vi "network_ping.vi"() -> ()   [LabVIEW 2011]
doc: "Use this template to build a standard state machine design pattern. Each state executes code and determines which state to transition to. Contrast this design pattern with the User Interface Event Handler pattern, in which code executes in response to user actions. Contrast this design pattern also with the Queued Message Handler pattern, in which each message handling code can queue zero or more new messages."
uses:
  StateMachineStates_ping.ctl
panel:
  out "RoundtripTime":i64
  out "Status":i32(ring) items=["Success"=0, "DestinationNetworkUnreachable"=11002, "DestinationHostUnreachable"=11003, "DestinationProhibited, DestinationProtocolUnreachable"=11004, "DestinationPortUnreachable"=11005, "NoResources"=11006, "BadOption"=11007, "HardwareError"=11008, "PacketTooBig"=11009, "TimedOut"=11010, "BadRoute"=11012, "TtlExpired"=11013, "TtlReassemblyTimeExceeded"=11014, "ParameterProblem"=11015, "SourceQuench"=11016, "BadDestination"=11018, "DestinationUnreachable"=11040, "TimeExceeded"=11041, "BadHeader"=11042, "UnrecognizedNextHeader"=11043, "IcmpError"=11044, "DestinationScopeMismatch"=11045, "Unknown"=-1]
  in  "hostNameOrAddress":string="127.0.0.1"
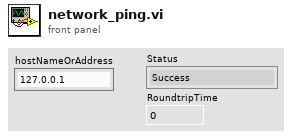
[diagram p1: front panel]
types:
  T1 = typedef "StateMachineStates_ping.ctl" = enum16{"Initialize", "ping_ok", "no_ping", "email", "Stop"}
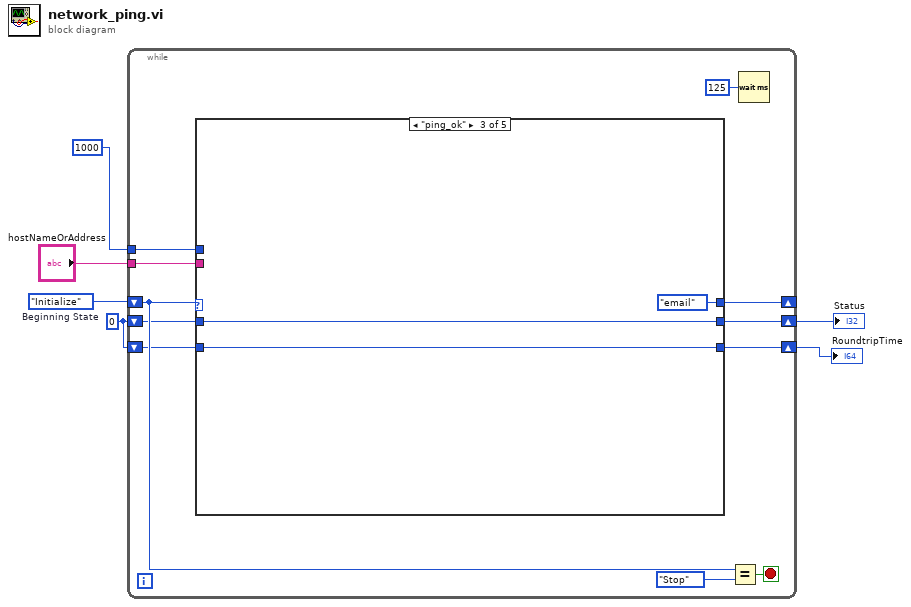
[diagram p0: block diagram]
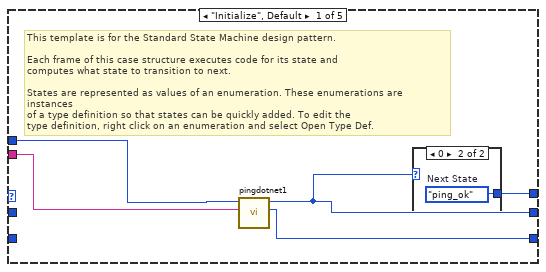
[diagram p2: hidden frame]
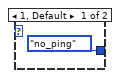
[diagram p3: hidden frame]
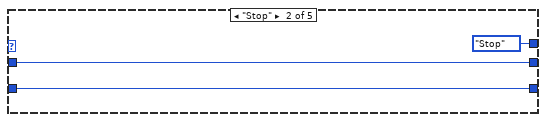
[diagram p4: hidden frame]
diagram:
  w1 = 0 ("Status")
  w6 = StateMachineStates_ping."Initialize"  # Beginning State
  n1 = while {
    shift-right: [w14] -> _
    shift-left: w6 -> [w15]
    tunnel: 1000 ("timeout") -> [w12]
    tunnel: "hostNameOrAddress" -> [w11]
    shift-right: [w10] -> w3
    shift-left: w1 -> [w9]
    shift-right: [w8] -> w2
    shift-left: w1 -> [w7]
    stop <- w17 stop-if-true
    n2 = case shown="\"ping_ok\"" w15 {
      tunnel: [w22 StateMachineStates_ping."Stop" ("Next State") StateMachineStates_ping."email" ("Next State") _ _] -> w14
      tunnel: w12 -> [w21 _ _ _ _]
      tunnel: w11 -> [w20 _ _ _ _]
      tunnel: [w18 w26 w29 _ _] -> w10
      tunnel: w9 -> [_ w26 w29 _ _]
      tunnel: [w19 w25 w30 _ _] -> w8
      tunnel: w7 -> [_ w25 w30 _ _]
      frame "Initialize", Default {
        # "This template is for the Standard State Machine design pattern.\n\nEach frame of this case structure executes code for its state and\ncomputes what state to transition to next.\n\nStates are represented as values of an enumeration. These enumerations are instances\nof a type definition so that states can be quickly added. To edit the \ntype definition, right click on an enumeration and select Open Type Def."
        n3 = call "pingdotnet1.vi"("hostNameOrAddress"=w20, "timeout"=w21) -> ("RoundtripTime"=w19:i64, "Status"=w18:i32)  [unwired: 4 in]
        n4 = case shown="0" w18 {
          tunnel: [StateMachineStates_ping."no_ping" ("Next State") w24] -> w22
          frame 1, Default {
          }
          frame 0 {
            w24 = StateMachineStates_ping."ping_ok"  # Next State
          }
        }
      }
      frame "Stop" {
      }
      frame "ping_ok" {
      }
      frame "no_ping" {
      }
      frame "email" {
      }
    }
    n5 = Equal?(x=w15, y=StateMachineStates_ping."Stop" ("States")) -> (x = y?=w17:bool)
    n6 = Wait (ms)(milliseconds to wait=u32 125) -> ()  [unwired: 1 out]
  }
  "Status" <- w3
  "RoundtripTime" <- w2
